vi "Compute DistanceToTarget With Angles.vi"(8 "Y Image Resolution":i32, 9 "X Image Resolution":i32, 10 "Vertical Strip":T1, 11 "Camera Type":enum16{"206", "1011", "1013"}(ring)) -> (0 "Center Displacement (ft)":dbl, 1 "Target Center (Angles)":cluster{dbl, dbl}, 2 "Target Center (-1 to 1)":cluster{"X":dbl, "Y":dbl}, 3 "Distance (ft)":dbl)   [LabVIEW 2013]
doc: "Using the camera lens information and the real world size of the target, use trig and ratios to determine the distance to the target. Also returns the location relative to the image center in a (-1 , 1) coordinate system that may be useful for steering the robot."
panel:
  in  "Camera view angles":dbl[](array[numeric])=[41.7, 37.4, 49.0]
  # "Axis 206\nAxis M1011\nAxis M1013"
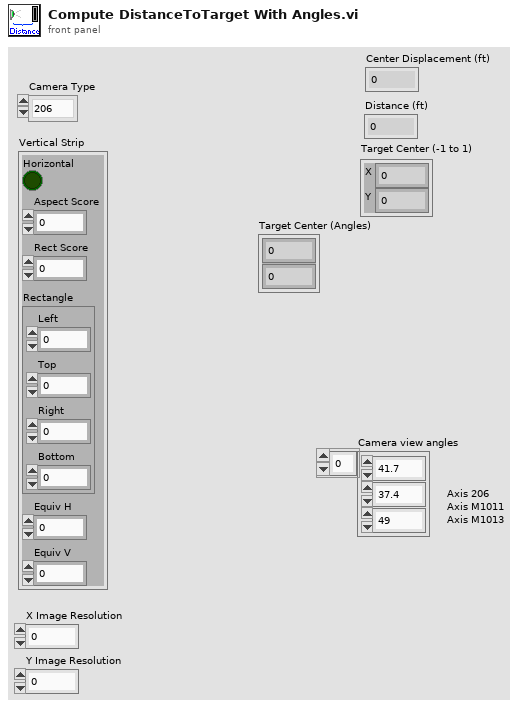
[diagram p1: front panel]
types:
  T1 = cluster{"Horizontal":bool, "Aspect Score":dbl, "Rect Score":dbl, "Rectangle":cluster{"Left":dbl, "Top":dbl, "Right":dbl, "Bottom":dbl}, "Equiv H":dbl, "Equiv V":dbl}
  T2 = cluster{"X Image Resolution":i32, "Y Image Resolution":i32}
  T3 = cluster{"X Image Resolution":dbl, "Y Image Resolution":dbl}
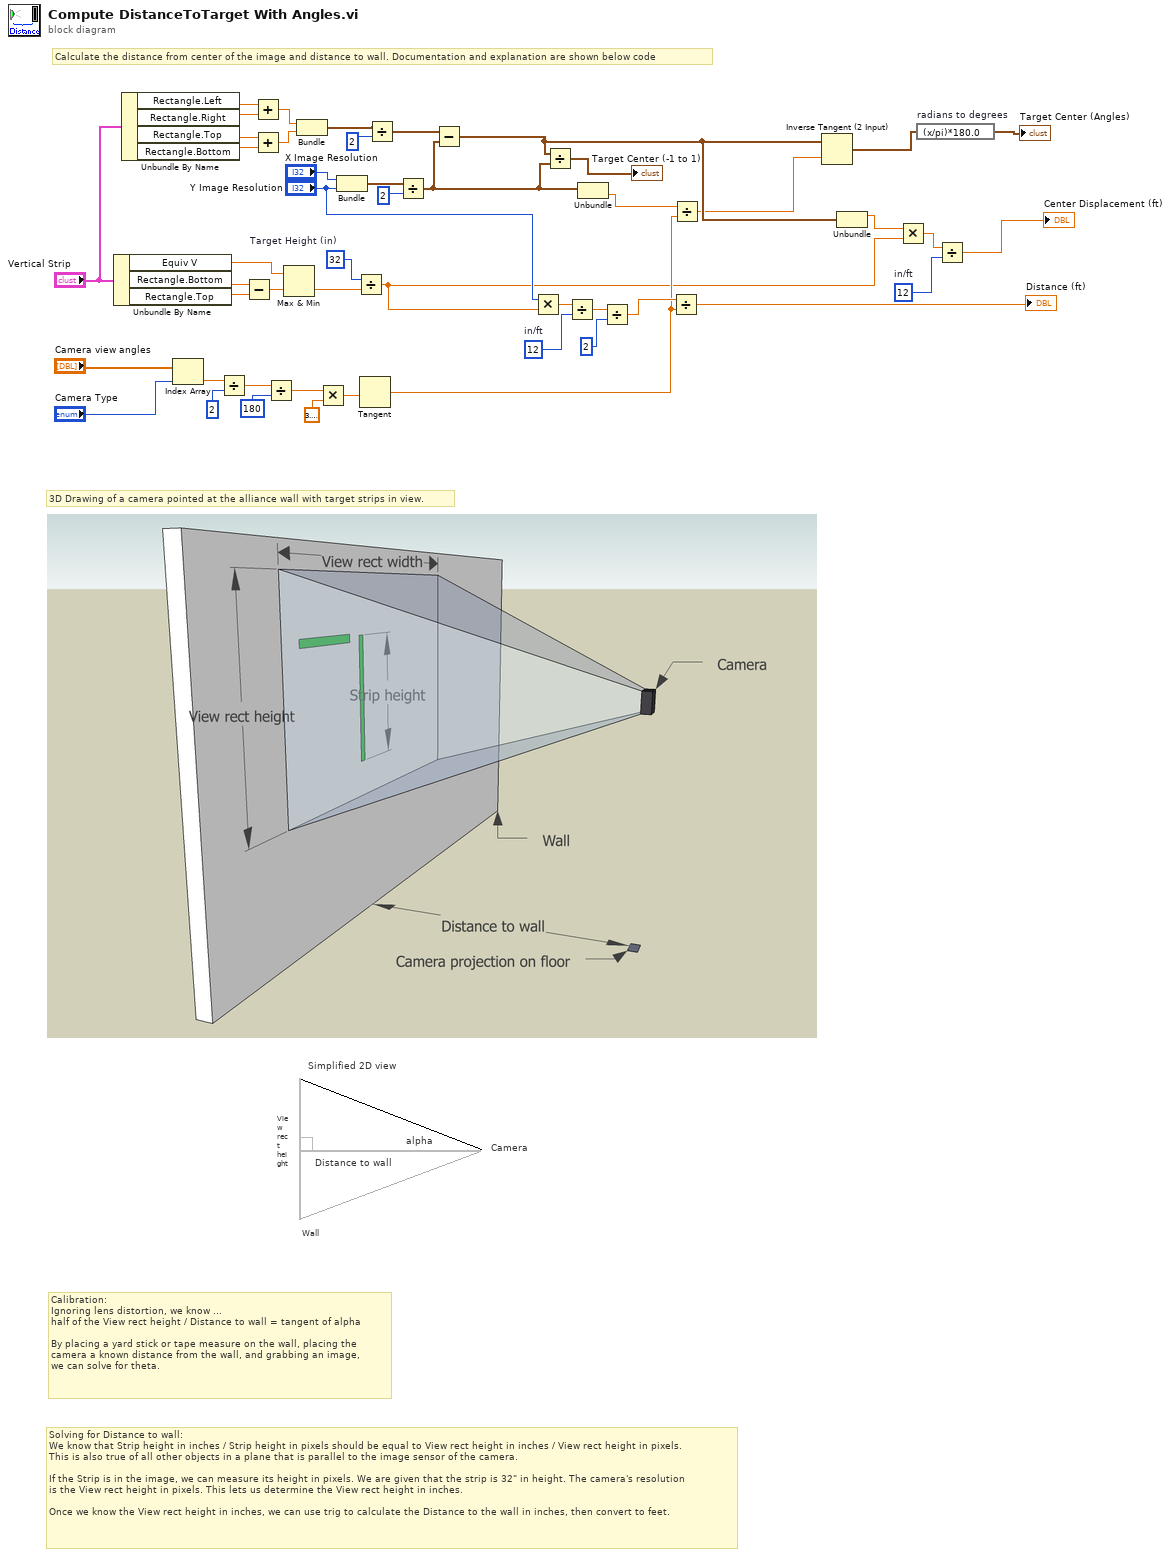
[diagram p0: block diagram]
diagram:
  w3 = 12  # in/ft
  w18 = 12  # in/ft
  w21 = 32  # Target Height (in)
  # "Wall"
  # "Camera"
  # "Simplified 2D view"
  # "Solving for Distance to wall:\nWe know that Strip height in inches / Strip height in pixels should be equal to View rect height in inches / View rect height in pixels.\nThis is also true of all other objects in a plane that is parallel to the image sensor of the camera.\n\nIf the Strip is in the image, we can measure its height in pixels. We are given that the strip is 32\" in height. The camera's resolution\nis the View rect height in pixels. This lets us determine the View rect height in inches.\n\nOnce we know the View rect height in inches, we can use trig to calculate the Distance to the wall in inches, then convert to feet."
  # "3D Drawing of a camera pointed at the alliance wall with target strips in view."
  # "Distance to wall"
  # "View rect height"
  # "alpha"
  # "Calibration:\nIgnoring lens distortion, we know ...\nhalf of the View rect height / Distance to wall = tangent of alpha\n\nBy placing a yard stick or tape measure on the wall, placing the\ncamera a known distance from the wall, and grabbing an image,\nwe can solve for theta."
  # "Calculate the distance from center of the image and distance to wall. Documentation and explanation are shown below code"
  n1 = Unbundle By Name("Vertical Strip") -> ("Equiv V"=w24:dbl, "Rectangle.Bottom"=w39:dbl, "Rectangle.Top"=w38:dbl)
  n2 = Unbundle By Name("Vertical Strip") -> ("Rectangle.Left"=w33:dbl, "Rectangle.Right"=w34:dbl, "Rectangle.Top"=w36:dbl, "Rectangle.Bottom"=w35:dbl)
  n3 = Index Array(array="Camera view angles", index="Camera Type") -> (element=w45:dbl)
  n4 = Divide(x=w45, y=2) -> (x/y=w42:dbl)
  n5 = Subtract(x=w39, y=w38) -> (x-y=w23:dbl)
  n6 = Add(x=w33, y=w34) -> (x+y=w31:dbl)
  n7 = Add(x=w36, y=w35) -> (x+y=w30:dbl)
  n8 = Divide(x=w42, y=180) -> (x/y=w41:dbl)
  n9 = Max & Min(x=w24, y=w23) -> (min(x,y)=w20:dbl)  [unwired: 1 out]
  n10 = Bundle(w31, w30) -> (w27:cluster{dbl, dbl})  [unwired: 1 in]
  n11 = Multiply(x=w41, y=3.141592653589793) -> (x*y=w43:dbl)
  n12 = Bundle("X Image Resolution"="X Image Resolution", "Y Image Resolution"="Y Image Resolution") -> (w29:T2)  [unwired: 1 in]
  n13 = Divide(x=w21, y=w20) -> (x/y=w4:dbl)
  n14 = Tangent(1:w43) -> (0:w11:dbl)
  n15 = Divide(x=w27, y=2) -> (x/y=w26:cluster{dbl, dbl})
  n16 = Divide(x=w29, y=2) -> (x/y=w12:T3)
  n17 = Subtract(x=w26, y=w12) -> (x-y=w7:cluster{dbl, dbl})
  n18 = Multiply(x="Y Image Resolution", y=w4) -> (x*y=w19:dbl)
  n19 = Divide(x=w7, y=w12) -> (x/y=→"Target Center (-1 to 1)":cluster{dbl, dbl})
  n20 = Divide(x=w19, y=w18) -> (x/y=w17:dbl)
  n21 = Unbundle(w12) -> ("Y Image Resolution"=w10:dbl)  [unwired: 1 out]
  n22 = Divide(x=w17, y=2) -> (x/y=w15:dbl)
  n23 = Divide(x=w15, y=w11) -> (x/y=→"Distance (ft)":dbl)
  n24 = Divide(x=w10, y=w11) -> (x/y=w6:dbl)
  n25 = Inverse Tangent (2 Input)(1:w6, 2:w7) -> (0:w9:cluster{dbl, dbl})
  n26 = Unbundle(w7) -> (w5:dbl)  [unwired: 1 out]
  n27 = Multiply(x=w5, y=w4) -> (x*y=w2:dbl)
  n28 = expression code="(x/pi)*180.0" "radians to degrees"(w9) -> (→"Target Center (Angles)":cluster{dbl, dbl})
  n29 = Divide(x=w2, y=w3) -> (x/y=→"Center Displacement (ft)":dbl)
